vi "Pump Out Selection.vi"(6 "Module Type":enum16{"Feed Module", "Pump Module"}(ring), 7 "Calibration Y Intercept":dbl, 8 "error in (no error)":errorcluster, 9 "Calibration Slope":dbl, 10 "Speed":dbl, 11 "Pump Settings In":T1={"Output Device"=enum."Default", "Masterflex"={"VISA resource name"="", "Simulated?"=FALSE, "Pump Number"=0.0, "Reverse?"=FALSE}, "Ismatech"={"VISA resource name"="", "Simulated?"=FALSE, "Pump Number"=0.0, "Reverse?"=FALSE}, "Ismatech 3 Channel Settings"={"VISA resource name"="", "Pump Number"=1, "Channel Number"=0, "Simulated?"=TRUE, "Reverse?"=FALSE}, "VICI Settings"={"VISA resource name"="", "Pump ID"="", "Pump Head Vol"=0.0, "Reverse?"=FALSE, "Simulated?"=FALSE}, "Tacmina Settings"={"Analog DAQ Task"="", "Digital DAQ Task"=""}, "KNF SIMDOS Settings"={"VISA resource name"="", "Simulated?"=FALSE}, "ASIA Pump C"={"ASIA Pump #"=0, "channel"=0, "Simulated"=FALSE}, "FLOM Settings"={"VISA resource name"="", "Simulated?"=FALSE, "Pump Number"=0.0}, "SSI PR/LD Settings"={"VISA resource name"="", "Simulated?"=FALSE}, "SSI P40 Settings"={"VISA resource name"="", "Simulated?"=FALSE}, "Masterflex 75211 Settings"={"Analog DAQ Task"="", "Digital DAQ Task"=""}} {"Ismatech 3 Channel Settings"."Channel Number" min=0 max=3; "Ismatech 3 Channel Settings"."Pump Number" min=1; "Masterflex"."Pump Number" min=1.0 max=20.0 step=1.0; "Ismatech"."Pump Number" min=1.0 max=20.0 step=1.0; "ASIA Pump C"."channel" min=-1 max=1 step=1}) -> (0 "error out":errorcluster, 2 "Connection Error":bool, 3 "Pump Settings Out":T1={"Output Device"=enum."Default", "Masterflex"={"VISA resource name"="", "Simulated?"=FALSE, "Pump Number"=0.0, "Reverse?"=FALSE}, "Ismatech"={"VISA resource name"="", "Simulated?"=FALSE, "Pump Number"=0.0, "Reverse?"=FALSE}, "Ismatech 3 Channel Settings"={"VISA resource name"="", "Pump Number"=1, "Channel Number"=0, "Simulated?"=TRUE, "Reverse?"=FALSE}, "VICI Settings"={"VISA resource name"="", "Pump ID"="", "Pump Head Vol"=0.0, "Reverse?"=FALSE, "Simulated?"=FALSE}, "Tacmina Settings"={"Analog DAQ Task"="", "Digital DAQ Task"=""}, "KNF SIMDOS Settings"={"VISA resource name"="", "Simulated?"=FALSE}, "ASIA Pump C"={"ASIA Pump #"=0, "channel"=0, "Simulated"=FALSE}, "FLOM Settings"={"VISA resource name"="", "Simulated?"=FALSE, "Pump Number"=0.0}, "SSI PR/LD Settings"={"VISA resource name"="", "Simulated?"=FALSE}, "SSI P40 Settings"={"VISA resource name"="", "Simulated?"=FALSE}, "Masterflex 75211 Settings"={"Analog DAQ Task"="", "Digital DAQ Task"=""}} {"Ismatech 3 Channel Settings"."Channel Number" min=0 max=3; "Ismatech 3 Channel Settings"."Pump Number" min=1; "Masterflex"."Pump Number" min=1.0 max=20.0 step=1.0; "Ismatech"."Pump Number" min=1.0 max=20.0 step=1.0; "ASIA Pump C"."channel" min=-1 max=1 step=1})   [LabVIEW 2018, in "Pump Module.lvlib" / "Pump Module Engine.lvlib"]
uses:
  Pump Module Engine.lvlib
  Pump Settings Cluster.ctl
  Measure Instrument/PID 2 Output Enum.ctl
  Masterflex 7550-30/Controls/Settings Cluster.ctl
  Ismatec ISM 831C/Controls/Ismatech ISM831C Settings Cluster.ctl
  Ismatec 78001/Ismatec 4083.ctl
  VICI M50 Party Mode/Settings Cluster.ctl
  Tacmina QI/Tacmina QI DAQ Setting.ctl
  KNF Pump/Settings Cluster plus SIMDOS.ctl
  ASIA Pump/Pump Settings.ctl
  FLOM Pump/Settings Cluster.ctl
  SSI PR Class/SSI PR or LD Settings Cluster.ctl
  Masterflex 75211/Masterflex 75211 DAQ Setting.ctl
  Ismatec ISM 831C/Ismatec ISM 831C.lvlib
  Masterflex 7550-30/Masterflex 7550-30.lvlib
  VICI M50 Party Mode/VICI M6 M50 Party Mode.lvlib
  Tacmina QI/Tacmina QI.lvlib
  KNF Pump/KNF SIMDOS.lvlib
  ASIA Pump.lvlib
  FLOM Pump/FLOM Pump.lvlib
  SSI PR Class/SSI PR or LD Pump.lvlib
  Masterflex 75211/Masterflex 75211.lvlib
  SSI PR Class/SSI P40 Pump.lvlib
  Ismatec 78001/Ismatec 4308.lvlib
  Pump Module.lvlib
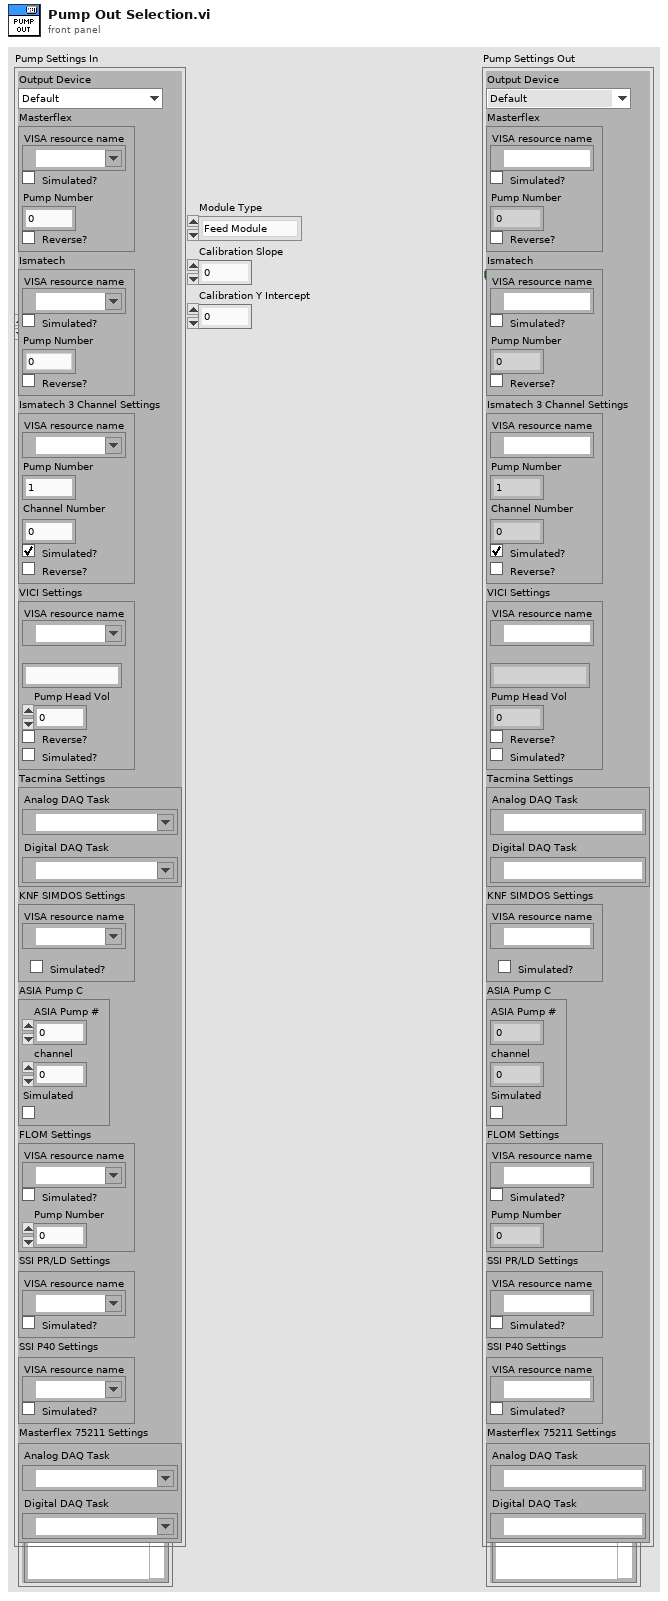
[diagram p1: front panel]
types:
  T1 = typedef "Pump Module.lvlib/Pump Settings Cluster.ctl" = cluster{"Output Device":T2, "Masterflex":T3, "Ismatech":T4, "Ismatech 3 Channel Settings":T5, "VICI Settings":T6, "Tacmina Settings":T7, "KNF SIMDOS Settings":T8, "ASIA Pump C":T9, "FLOM Settings":T10, "SSI PR/LD Settings":T11, "SSI P40 Settings":T11, "Masterflex 75211 Settings":T12}
  T2 = typedef "PID 2 Output Enum.ctl" = enum16{"Default", "Ismatec ISM 4308", "Ismatec ISM 831C", "Masterflex 7550-30", "VICI M6", "VICI M50", "Tacmina QI", "KNF SIMDOS", "ASIA Type C", "FLOM UI-22-11", "SSI PR/LD", "SSI P40", "Masterflex 75211-70"}
  T3 = typedef "Masterflex 7550-30.lvlib/Settings Cluster.ctl" = cluster{"VISA resource name":refnum<visa-resource-name>, "Simulated?":bool, "Pump Number":dbl, "Reverse?":bool}
  T4 = typedef "Ismatec ISM 831C.lvlib/Ismatech ISM831C Settings Cluster.ctl" = cluster{"VISA resource name":refnum<visa-resource-name>, "Simulated?":bool, "Pump Number":dbl, "Reverse?":bool}
  T5 = typedef "Ismatec 4308.lvlib/Ismatec 4083.ctl" = cluster{"VISA resource name":refnum<visa-resource-name>, "Pump Number":i16, "Channel Number":i16, "Simulated?":bool, "Reverse?":bool}
  T6 = typedef "VICI M6 M50 Party Mode.lvlib/Settings Cluster.ctl" = cluster{"VISA resource name":refnum<visa-resource-name>, "Pump ID":string, "Pump Head Vol":dbl, "Reverse?":bool, "Simulated?":bool}
  T7 = typedef "Tacmina QI.lvlib/Tacmina QI DAQ Setting.ctl" = cluster{"Analog DAQ Task":refnum<k21>, "Digital DAQ Task":refnum<k21>}
  T8 = typedef "KNF SIMDOS.lvlib/Settings Cluster plus SIMDOS.ctl" = cluster{"VISA resource name":refnum<visa-resource-name>, "Simulated?":bool}
  T9 = typedef "ASIA Pump.lvlib/Pump Settings.ctl" = cluster{"ASIA Pump #":i32, "channel":i32, "Simulated":bool}
  T10 = typedef "FLOM Pump.lvlib/Settings Cluster.ctl" = cluster{"VISA resource name":refnum<visa-resource-name>, "Simulated?":bool, "Pump Number":dbl}
  T11 = typedef "SSI PR or LD Pump.lvlib/SSI PR or LD Settings Cluster.ctl" = cluster{"VISA resource name":refnum<visa-resource-name>, "Simulated?":bool}
  T12 = typedef "Masterflex 75211.lvlib/Masterflex 75211 DAQ Setting.ctl" = cluster{"Analog DAQ Task":refnum<k21>, "Digital DAQ Task":refnum<k21>}
  T13 = typedef "SSI P40 Pump.lvlib/SSI P40 Settings Cluster.ctl" = cluster{"VISA resource name":refnum<visa-resource-name>, "Simulated?":bool}
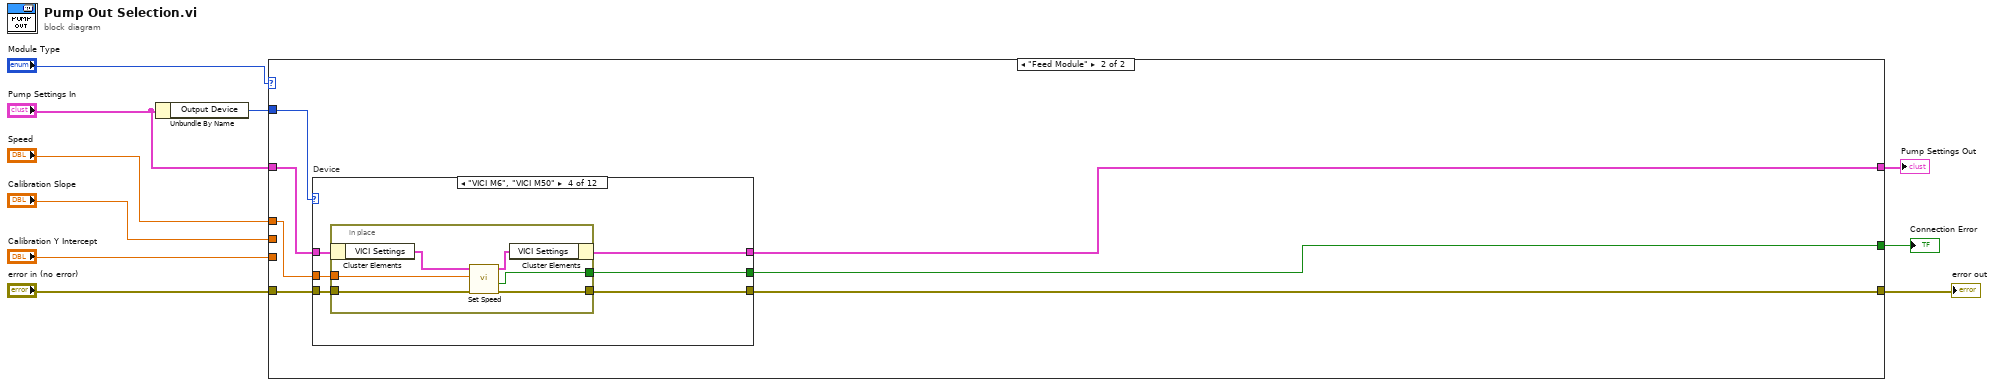
[diagram p0: block diagram]
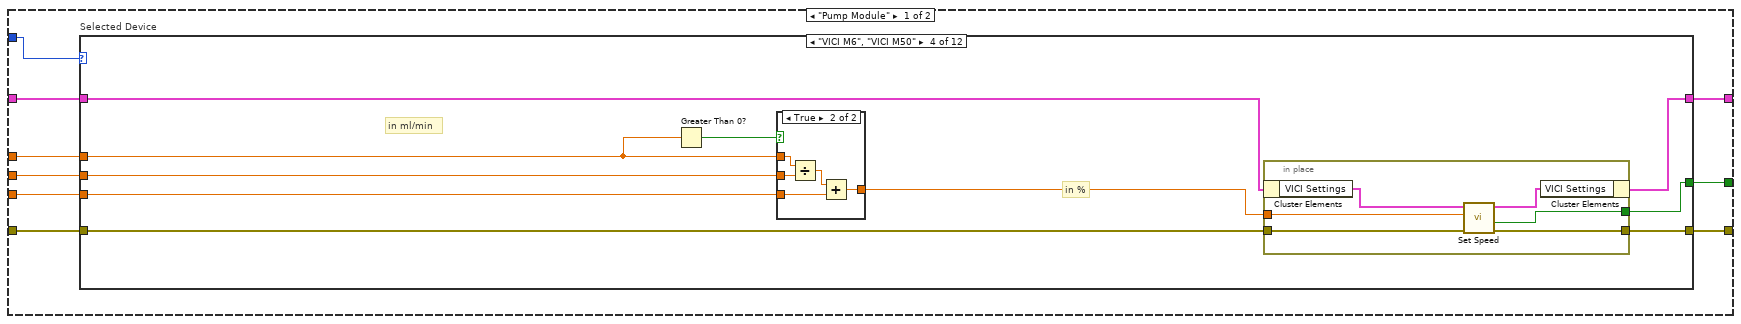
[diagram p2: hidden frame]
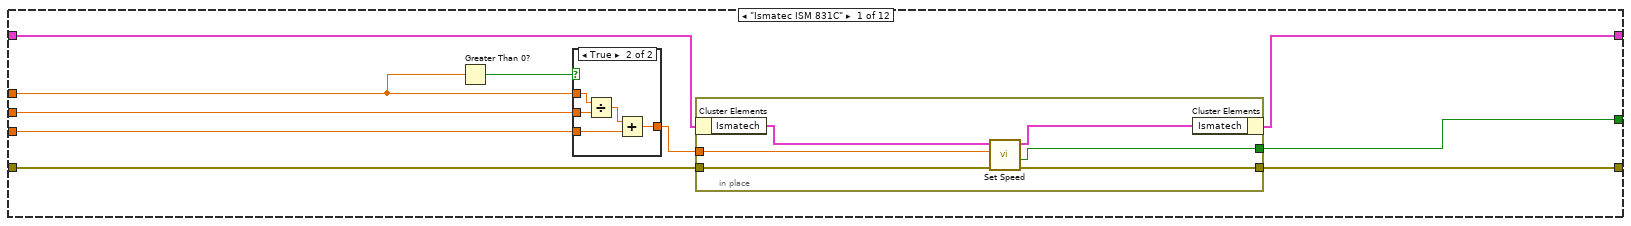
[diagram p3: hidden frame]
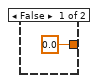
[diagram p4: hidden frame]
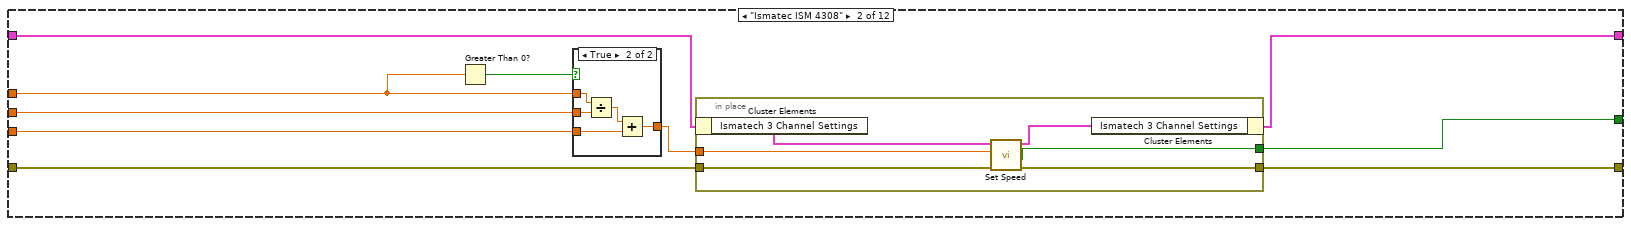
[diagram p5: hidden frame]
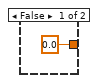
[diagram p6: hidden frame]
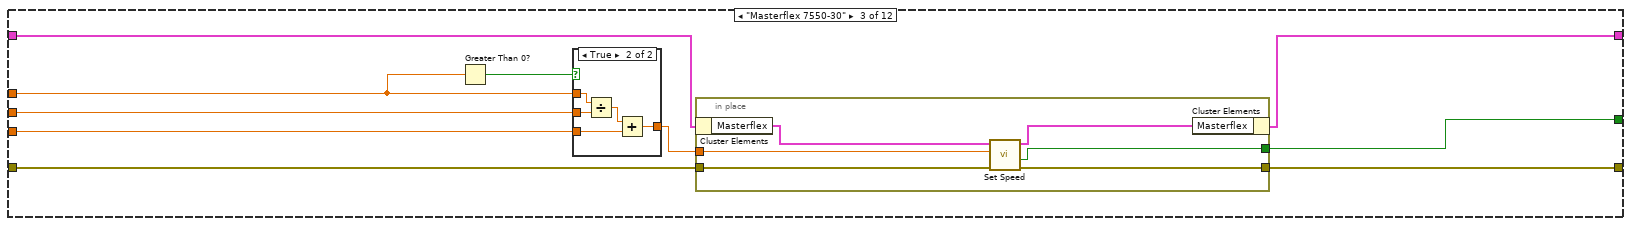
[diagram p7: hidden frame]
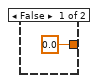
[diagram p8: hidden frame]
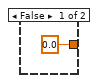
[diagram p9: hidden frame]
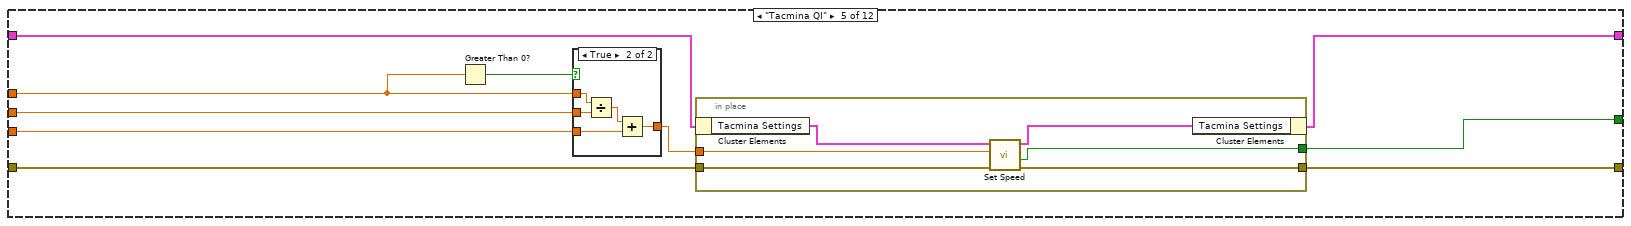
[diagram p10: hidden frame]
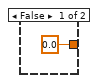
[diagram p11: hidden frame]
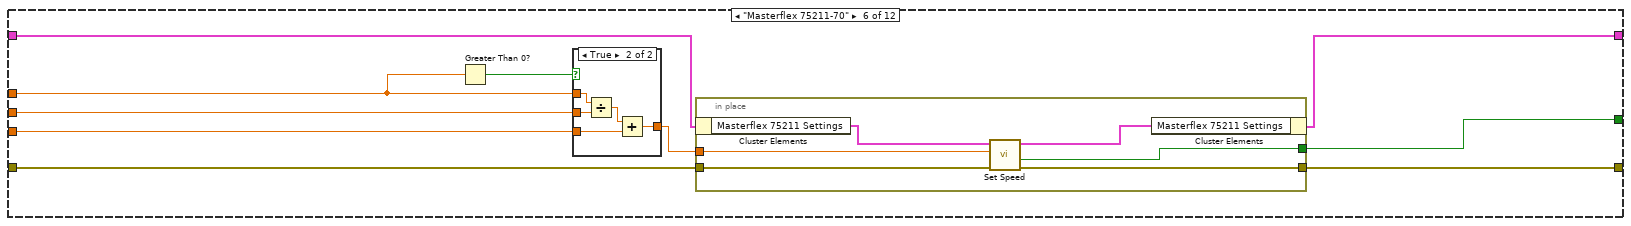
[diagram p12: hidden frame]
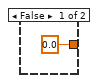
[diagram p13: hidden frame]
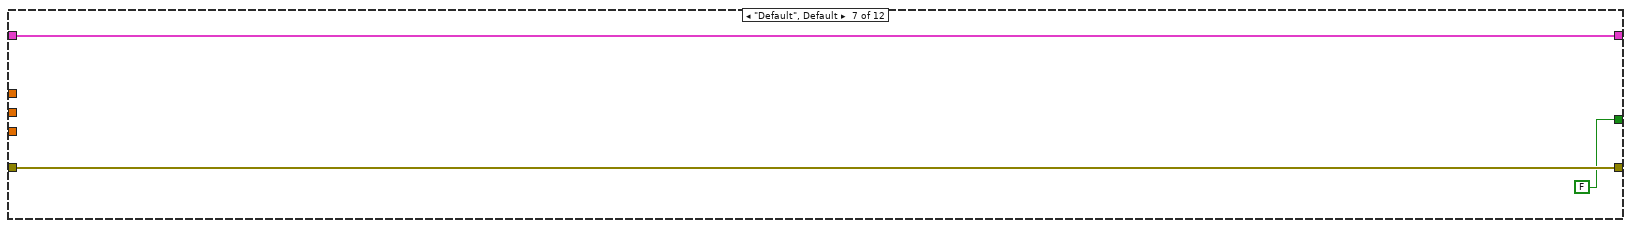
[diagram p14: hidden frame]
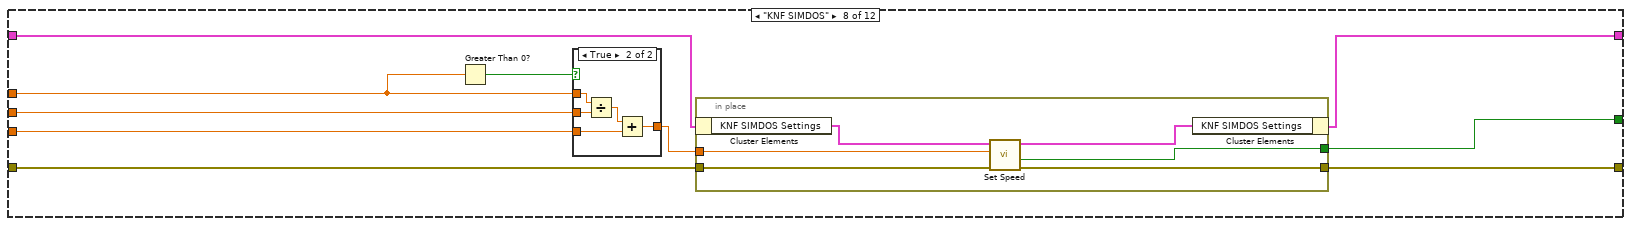
[diagram p15: hidden frame]
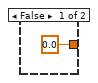
[diagram p16: hidden frame]
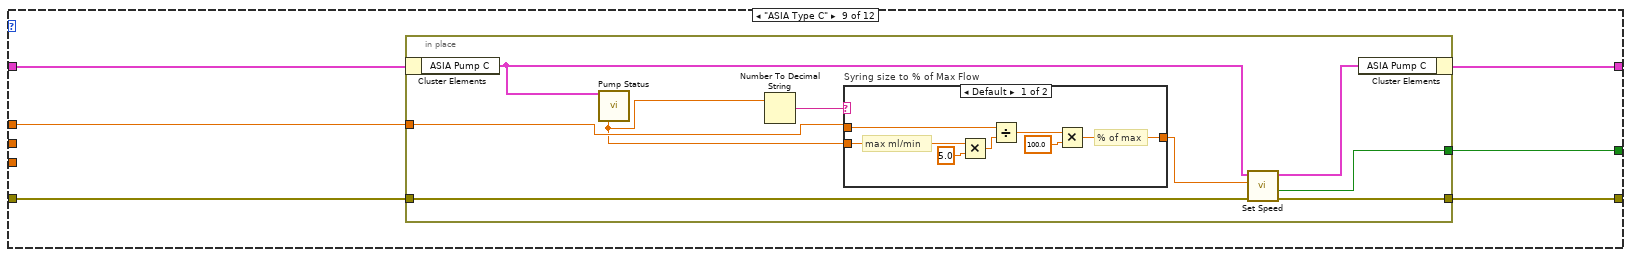
[diagram p17: hidden frame]
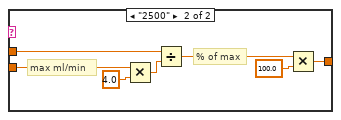
[diagram p18: hidden frame]
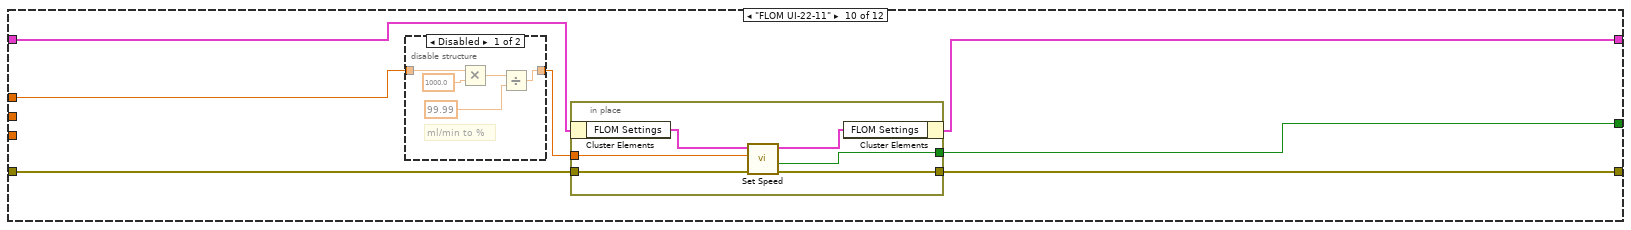
[diagram p19: hidden frame]
diagram:
  n1 = Unbundle By Name("Pump Settings In") -> ("Output Device"=w5:T2)
  n2 = case shown="\"Feed Module\"" "Module Type" {
    tunnel: [w19 w251] -> w10
    tunnel: [w18 w250] -> w9
    tunnel: "error in (no error)" -> [w17 w254]
    tunnel: "Speed" -> [w16 w253]
    tunnel: [w15 w252] -> w3
    tunnel: w5 -> [w14 w255]
    tunnel: "Calibration Slope" -> [w13 _]
    tunnel: "Calibration Y Intercept" -> [w12 _]
    tunnel: "Pump Settings In" -> [w11 w249]
    frame "Pump Module" {
      n3 = case "Selected Device" shown="\"VICI M6\", \"VICI M50\"" w14 {
        tunnel: w16 -> [w23 w45 w69 w91 w113 w135 _ w160 w179 w208 w230 w242]
        tunnel: w17 -> [w29 w51 w73 w95 w117 w139 w154 w164 w182 w212 w228 w240]
        tunnel: [w28 w50 w72 w94 w116 w138 w154 w163 w181 w210 w229 w241] -> w18
        tunnel: [w20 w42 w64 w86 w108 w130 w152 w155 w177 w206 w225 w237] -> w15
        tunnel: [w27 w49 w71 w93 w115 w137 FALSE ("Connection Error") w162 w180 w211 w227 w239] -> w19
        tunnel: w13 -> [w25 w47 w67 w90 w112 w134 _ w159 _ _ _ _]
        tunnel: w12 -> [w26 w48 w68 w88 w111 w133 _ w158 _ _ _ _]
        tunnel: w11 -> [w21 w43 w65 w87 w109 w131 w152 w156 w178 w207 w226 w238]
        frame "Ismatec ISM 831C" {
          n4 = Greater Than 0?(x=w23) -> (x > 0?=w22:bool)
          n5 = case shown="True" w22 {
            tunnel: w26 -> [_ w40]
            tunnel: w25 -> [_ w39]
            tunnel: w23 -> [_ w38]
            tunnel: [0.0 w37] -> w24
            frame False {
            }
            frame True {
              n6 = Divide(x=w38, y=w39) -> (x/y=w41:dbl)
              n7 = Add(x=w41, y=w40) -> (x+y=w37:dbl)
            }
          }
          n8 = in-place {
            in-place-border: w29 -> [w35]
            in-place-border: [w34] -> w28
            in-place-border: [w33] -> w27
            in-place-border: w24 -> [w32]
            n9 = in-place-cluster #1(w21) -> ("Ismatech"=w31:T4)
            n10 = call "Set Speed.vi"("error in (no error)"=w35, "Speed (%)"=w32, "Ismatech Settings In"=w31) -> ("error out"=w34:errorcluster, "Connection Error"=w33:bool, "Ismatech Settings Out"=w30:T4)  [unwired: 6 in]
            n11 = in-place-cluster #1("Ismatech"=w30) -> (w20:T1)
          }
        }
        frame "Ismatec ISM 4308" {
          n12 = Greater Than 0?(x=w45) -> (x > 0?=w44:bool)
          n13 = case shown="True" w44 {
            tunnel: w48 -> [_ w62]
            tunnel: w47 -> [_ w61]
            tunnel: w45 -> [_ w60]
            tunnel: [0.0 w59] -> w46
            frame False {
            }
            frame True {
              n14 = Divide(x=w60, y=w61) -> (x/y=w63:dbl)
              n15 = Add(x=w63, y=w62) -> (x+y=w59:dbl)
            }
          }
          n16 = in-place {
            in-place-border: w51 -> [w55]
            in-place-border: [w54] -> w50
            in-place-border: [w53] -> w49
            in-place-border: w46 -> [w56]
            n17 = in-place-cluster #2(w43) -> ("Ismatech 3 Channel Settings"=w57:T5)
            n18 = call "Set Speed.vi"("error in (no error)"=w55, "Speed (%)"=w56, "Ismatech 3 Channel Settings In"=w57) -> ("error out"=w54:errorcluster, "Connection Error"=w53:bool, "Ismatech 3 Channel Settings Out"=w52:T5)  [unwired: 5 in, 1 out]
            n19 = in-place-cluster #2("Ismatech 3 Channel Settings"=w52) -> (w42:T1)
          }
        }
        frame "Masterflex 7550-30" {
          n20 = Greater Than 0?(x=w69) -> (x > 0?=w70:bool)
          n21 = case shown="True" w70 {
            tunnel: w68 -> [_ w84]
            tunnel: w67 -> [_ w83]
            tunnel: w69 -> [_ w82]
            tunnel: [0.0 w81] -> w66
            frame False {
            }
            frame True {
              n22 = Divide(x=w82, y=w83) -> (x/y=w85:dbl)
              n23 = Add(x=w85, y=w84) -> (x+y=w81:dbl)
            }
          }
          n24 = in-place {
            in-place-border: w73 -> [w79]
            in-place-border: [w78] -> w72
            in-place-border: [w77] -> w71
            in-place-border: w66 -> [w76]
            n25 = in-place-cluster #3(w65) -> ("Masterflex"=w75:T3)
            n26 = call "Set Speed.vi"("error in (no error)"=w79, "speed"=w76, "Masterflex Settings in"=w75) -> ("error out"=w78:errorcluster, "Connection Error"=w77:bool, "Masterflex Settings out"=w74:T3)  [unwired: 6 in]
            n27 = in-place-cluster #3("Masterflex"=w74) -> (w64:T1)
          }
        }
        frame "VICI M6", "VICI M50" {
          # "in ml/min"
          # "in %"
          n28 = Greater Than 0?(x=w91) -> (x > 0?=w92:bool)
          n29 = case shown="True" w92 {
            tunnel: w88 -> [_ w106]
            tunnel: w90 -> [_ w105]
            tunnel: w91 -> [_ w104]
            tunnel: [0.0 w103] -> w89
            frame False {
            }
            frame True {
              n30 = Divide(x=w104, y=w105) -> (x/y=w107:dbl)
              n31 = Add(x=w107, y=w106) -> (x+y=w103:dbl)
            }
          }
          n32 = in-place {
            in-place-border: w95 -> [w101]
            in-place-border: [w100] -> w94
            in-place-border: [w99] -> w93
            in-place-border: w89 -> [w98]
            n33 = in-place-cluster #4(w87) -> ("VICI Settings"=w96:T6)
            n34 = call "Set Speed.vi"("error in (no error)"=w101, "Flow Rate (mL/min)"=w98, "VICI Settings In"=w96) -> ("error out"=w100:errorcluster, "Connection Error"=w99:bool, "VICI Settings Out"=w97:T6)  [unwired: 6 in]
            n35 = in-place-cluster #4("VICI Settings"=w97) -> (w86:T1)
          }
        }
        frame "Tacmina QI" {
          n36 = Greater Than 0?(x=w113) -> (x > 0?=w114:bool)
          n37 = case shown="True" w114 {
            tunnel: w111 -> [_ w128]
            tunnel: w112 -> [_ w127]
            tunnel: w113 -> [_ w126]
            tunnel: [0.0 w125] -> w110
            frame False {
            }
            frame True {
              n38 = Divide(x=w126, y=w127) -> (x/y=w129:dbl)
              n39 = Add(x=w129, y=w128) -> (x+y=w125:dbl)
            }
          }
          n40 = in-place {
            in-place-border: w117 -> [w123]
            in-place-border: [w122] -> w116
            in-place-border: [w121] -> w115
            in-place-border: w110 -> [w120]
            n41 = in-place-cluster #5(w109) -> ("Tacmina Settings"=w119:T7)
            n42 = call "Set Speed.vi"("error in"=w123, "Pump %"=w120, "Tacmina Settings in"=w119) -> ("error out"=w122:errorcluster, "Connection Error"=w121:bool, "Tacmina Settings out"=w118:T7)  [unwired: 6 in]
            n43 = in-place-cluster #5("Tacmina Settings"=w118) -> (w108:T1)
          }
        }
        frame "Masterflex 75211-70" {
          n44 = Greater Than 0?(x=w135) -> (x > 0?=w136:bool)
          n45 = case shown="True" w136 {
            tunnel: w133 -> [_ w150]
            tunnel: w134 -> [_ w149]
            tunnel: w135 -> [_ w148]
            tunnel: [0.0 w147] -> w132
            frame False {
            }
            frame True {
              n46 = Divide(x=w148, y=w149) -> (x/y=w151:dbl)
              n47 = Add(x=w151, y=w150) -> (x+y=w147:dbl)
            }
          }
          n48 = in-place {
            in-place-border: w139 -> [w140]
            in-place-border: [w142] -> w138
            in-place-border: [w143] -> w137
            in-place-border: w132 -> [w141]
            n49 = in-place-cluster #6(w131) -> ("Masterflex 75211 Settings"=w145:T12)
            n50 = call "Set Speed.vi"("error in"=w140, "Pump %"=w141, "Masterflex 75211 Settings"=w145) -> ("error out"=w142:errorcluster, "Connection Error"=w143:bool, "Masterflex 75211 Settings 2"=w144:T12)  [unwired: 6 in]
            n51 = in-place-cluster #6("Masterflex 75211 Settings"=w144) -> (w130:T1)
          }
        }
        frame "Default", Default {
        }
        frame "KNF SIMDOS" {
          n52 = Greater Than 0?(x=w160) -> (x > 0?=w161:bool)
          n53 = case shown="True" w161 {
            tunnel: w158 -> [_ w175]
            tunnel: w159 -> [_ w174]
            tunnel: w160 -> [_ w173]
            tunnel: [0.0 w172] -> w157
            frame False {
            }
            frame True {
              n54 = Divide(x=w173, y=w174) -> (x/y=w176:dbl)
              n55 = Add(x=w176, y=w175) -> (x+y=w172:dbl)
            }
          }
          n56 = in-place {
            in-place-border: w164 -> [w170]
            in-place-border: [w169] -> w163
            in-place-border: [w168] -> w162
            in-place-border: w157 -> [w167]
            n57 = in-place-cluster #7(w156) -> ("KNF SIMDOS Settings"=w166:T8)
            n58 = call "Set Speed.vi"("error in (no error)"=w170, "FlowRate"=w167, "KNF Settings In"=w166) -> ("error out"=w169:errorcluster, "Connection Error"=w168:bool, "KNF Settings Out"=w165:T8)  [unwired: 6 in]
            n59 = in-place-cluster #7("KNF SIMDOS Settings"=w165) -> (w155:T1)
          }
        }
        frame "ASIA Type C" {
          n60 = in-place {
            in-place-border: w182 -> [w191]
            in-place-border: [w190] -> w181
            in-place-border: [w189] -> w180
            in-place-border: w179 -> [w188]
            n61 = in-place-cluster #8(w178) -> ("ASIA Pump C"=w183:T9)
            n62 = call "Pump Status.vi"("ASIA Pump C Settings in"=w183) -> ("syringeSize (ml)"=w185:sgl)  [unwired: 6 in, 8 out]
            n63 = Number To Decimal String(number=w185) -> (decimal integer string=w187:string)  [unwired: 1 in]
            n64 = case "Syring size to % of Max Flow" shown="Default" w187 {
              tunnel: w185 -> [w197 w201]
              tunnel: w188 -> [w196 w200]
              tunnel: [w192 w199] -> w186
              frame Default {
                # "% of max"
                # "max ml/min"
                n65 = Multiply(x=w197, y=5.0) -> (x*y=w195:dbl)
                n66 = Divide(x=w196, y=w195) -> (x/y=w194:dbl)
                n67 = Multiply(x=w194, y=100.0) -> (x*y=w192:dbl)
              }
              frame "2500" {
                # "% of max"
                # "max ml/min"
                n68 = Multiply(x=w201, y=4.0) -> (x*y=w204:dbl)
                n69 = Divide(x=w200, y=w204) -> (x/y=w203:dbl)
                n70 = Multiply(x=w203, y=100.0) -> (x*y=w199:dbl)
              }
            }
            n71 = call "Set Speed.vi"("error in (no error)"=w191, "Pump %"=w186, "ASIA Pump C Settings in"=w183) -> ("error out"=w190:errorcluster, "Connection Error"=w189:bool, "ASIA Pump C Settings out"=w184:T9)  [unwired: 6 in]
            n72 = in-place-cluster #8("ASIA Pump C"=w184) -> (w177:T1)
          }
        }
        frame "FLOM UI-22-11" {
          n73 = disable-structure shown="Disabled" {
            disable-tunnel: [w222 w224] -> w209
            disable-tunnel: w208 -> [w220 w224]
            frame Disabled {
              # "ml/min to %"
              n74 = Multiply(x=w220, y=1000.0) -> (x*y=w219:dbl)
              n75 = Divide(x=w219, y=99.99) -> (x/y=w222:dbl)
            }
            frame Enabled {
            }
          }
          n76 = in-place {
            in-place-border: w212 -> [w218]
            in-place-border: [w217] -> w211
            in-place-border: [w216] -> w210
            in-place-border: w209 -> [w215]
            n77 = in-place-cluster #9(w207) -> ("FLOM Settings"=w213:T10)
            n78 = call "Set Speed.vi"("error in (no error)"=w218, "speed"=w215, "FLOM Settings in"=w213) -> ("error out"=w216:errorcluster, "Connection Error"=w217:bool, "FLOM Settings out"=w214:T10)  [unwired: 6 in]
            n79 = in-place-cluster #9("FLOM Settings"=w214) -> (w206:T1)
          }
        }
        frame "SSI PR/LD" {
          n80 = in-place {
            in-place-border: w230 -> [w236]
            in-place-border: [w235] -> w229
            in-place-border: w228 -> [w234]
            in-place-border: [w233] -> w227
            n81 = in-place-cluster #10(w226) -> ("SSI PR/LD Settings"=w231:T11)
            n82 = call "Set Speed.vi"("error in (no error)"=w234, "speed (ml/min)"=w236, "SSI PR Settings In"=w231) -> ("error out"=w235:errorcluster, "Connection Error"=w233:bool, "SSI PR Settings Out"=w232:T11)  [unwired: 6 in]
            n83 = in-place-cluster #10("SSI PR/LD Settings"=w232) -> (w225:T1)
          }
        }
        frame "SSI P40" {
          n84 = in-place {
            in-place-border: w242 -> [w247]
            in-place-border: [w245] -> w241
            in-place-border: w240 -> [w246]
            in-place-border: [w244] -> w239
            n85 = in-place-cluster #11(w238) -> ("SSI P40 Settings"=w248:T11)
            n86 = call "Set Speed P40.vi"("error in (no error)"=w246, "speed (ml/min)"=w247, "SSI P40 Settings In"=w248) -> ("error out"=w245:errorcluster, "Connection Error"=w244:bool, "SSI P40 Settings Out"=w243:T13)  [unwired: 6 in]
            n87 = in-place-cluster #11("SSI P40 Settings"=w243) -> (w237:T1)
          }
        }
      }
    }
    frame "Feed Module" {
      n88 = case "Device" shown="\"VICI M6\", \"VICI M50\"" w255 {
        tunnel: w253 -> [w259 w271 w283 w297 w309 w321 _ w336 w348 w359 w370 w382]
        tunnel: w254 -> [w261 w273 w285 w296 w308 w320 w329 w335 w345 w360 w372 w384]
        tunnel: [w260 w272 w284 w295 w307 w319 w329 w334 w347 w357 w371 w383] -> w250
        tunnel: w249 -> [w257 w269 w281 w293 w305 w317 w330 w332 w344 w356 w368 w380]
        tunnel: [w256 w268 w280 w292 w304 w316 w330 w331 w343 w355 w367 w379] -> w252
        tunnel: [w258 w270 w282 w294 w306 w318 FALSE ("Connection Error") w333 w346 w358 w369 w381] -> w251
        frame "Ismatec ISM 831C" {
          n89 = in-place {
            in-place-border: w261 -> [w267]
            in-place-border: [w266] -> w260
            in-place-border: w257 -> [_]
            in-place-border: w259 -> [w265]
            in-place-border: [w264] -> w258
            n90 = in-place-cluster #12(w257) -> ("Ismatech"=w262:T4)
            n91 = call "Set Speed.vi"("error in (no error)"=w267, "Speed (%)"=w265, "Ismatech Settings In"=w262) -> ("error out"=w266:errorcluster, "Connection Error"=w264:bool, "Ismatech Settings Out"=w263:T4)  [unwired: 6 in]
            n92 = in-place-cluster #12("Ismatech"=w263) -> (w256:T1)
          }
        }
        frame "Ismatec ISM 4308" {
          n93 = in-place {
            in-place-border: w273 -> [w279]
            in-place-border: [w278] -> w272
            in-place-border: w271 -> [w275]
            in-place-border: [w274] -> w270
            n94 = in-place-cluster #13(w269) -> ("Ismatech 3 Channel Settings"=w276:T5)
            n95 = call "Set Speed.vi"("error in (no error)"=w279, "Speed (%)"=w275, "Ismatech 3 Channel Settings In"=w276) -> ("error out"=w278:errorcluster, "Connection Error"=w274:bool, "Ismatech 3 Channel Settings Out"=w277:T5)  [unwired: 5 in, 1 out]
            n96 = in-place-cluster #13("Ismatech 3 Channel Settings"=w277) -> (w268:T1)
          }
        }
        frame "Masterflex 7550-30" {
          n97 = in-place {
            in-place-border: w285 -> [w291]
            in-place-border: [w290] -> w284
            in-place-border: w283 -> [w289]
            in-place-border: [w288] -> w282
            n98 = in-place-cluster #14(w281) -> ("Masterflex"=w287:T3)
            n99 = call "Set Speed.vi"("error in (no error)"=w291, "speed"=w289, "Masterflex Settings in"=w287) -> ("error out"=w290:errorcluster, "Connection Error"=w288:bool, "Masterflex Settings out"=w286:T3)  [unwired: 6 in]
            n100 = in-place-cluster #14("Masterflex"=w286) -> (w280:T1)
          }
        }
        frame "VICI M6", "VICI M50" {
          n101 = in-place {
            in-place-border: w297 -> [w303]
            in-place-border: w296 -> [w302]
            in-place-border: [w301] -> w295
            in-place-border: [w300] -> w294
            n102 = in-place-cluster #15(w293) -> ("VICI Settings"=w298:T6)
            n103 = call "Set Speed.vi"("error in (no error)"=w302, "Flow Rate (mL/min)"=w303, "VICI Settings In"=w298) -> ("error out"=w301:errorcluster, "Connection Error"=w300:bool, "VICI Settings Out"=w299:T6)  [unwired: 6 in]
            n104 = in-place-cluster #15("VICI Settings"=w299) -> (w292:T1)
          }
        }
        frame "Tacmina QI" {
          n105 = in-place {
            in-place-border: w309 -> [w315]
            in-place-border: w308 -> [w314]
            in-place-border: [w313] -> w307
            in-place-border: [w312] -> w306
            n106 = in-place-cluster #16(w305) -> ("Tacmina Settings"=w310:T7)
            n107 = call "Set Speed.vi"("error in"=w314, "Pump %"=w315, "Tacmina Settings in"=w310) -> ("error out"=w313:errorcluster, "Connection Error"=w312:bool, "Tacmina Settings out"=w311:T7)  [unwired: 6 in]
            n108 = in-place-cluster #16("Tacmina Settings"=w311) -> (w304:T1)
          }
        }
        frame "Masterflex 75211-70" {
          n109 = in-place {
            in-place-border: w321 -> [w325]
            in-place-border: w320 -> [w326]
            in-place-border: [w322] -> w319
            in-place-border: [w323] -> w318
            n110 = in-place-cluster #17(w317) -> ("Masterflex 75211 Settings"=w327:T12)
            n111 = call "Set Speed.vi"("error in"=w326, "Pump %"=w325, "Masterflex 75211 Settings"=w327) -> ("error out"=w322:errorcluster, "Connection Error"=w323:bool, "Masterflex 75211 Settings 2"=w324:T12)  [unwired: 6 in]
            n112 = in-place-cluster #17("Masterflex 75211 Settings"=w324) -> (w316:T1)
          }
        }
        frame "Default", Default {
        }
        frame "KNF SIMDOS" {
          n113 = in-place {
            in-place-border: w336 -> [w342]
            in-place-border: w335 -> [w341]
            in-place-border: [w340] -> w334
            in-place-border: [w339] -> w333
            n114 = in-place-cluster #18(w332) -> ("KNF SIMDOS Settings"=w338:T8)
            n115 = call "Set Speed.vi"("error in (no error)"=w341, "FlowRate"=w342, "KNF Settings In"=w338) -> ("error out"=w340:errorcluster, "Connection Error"=w339:bool, "KNF Settings Out"=w337:T8)  [unwired: 6 in]
            n116 = in-place-cluster #18("KNF SIMDOS Settings"=w337) -> (w331:T1)
          }
        }
        frame "ASIA Type C" {
          n117 = in-place {
            in-place-border: w348 -> [w354]
            in-place-border: [w353] -> w347
            in-place-border: [w352] -> w346
            in-place-border: w345 -> [w351]
            n118 = in-place-cluster #19(w344) -> ("ASIA Pump C"=w350:T9)
            n119 = call "Set Speed.vi"("error in (no error)"=w351, "Pump %"=w354, "ASIA Pump C Settings in"=w350) -> ("error out"=w353:errorcluster, "Connection Error"=w352:bool, "ASIA Pump C Settings out"=w349:T9)  [unwired: 6 in]
            n120 = in-place-cluster #19("ASIA Pump C"=w349) -> (w343:T1)
          }
        }
        frame "FLOM UI-22-11" {
          n121 = in-place {
            in-place-border: w360 -> [w366]
            in-place-border: w359 -> [w365]
            in-place-border: [w364] -> w358
            in-place-border: [w363] -> w357
            n122 = in-place-cluster #20(w356) -> ("FLOM Settings"=w361:T10)
            n123 = call "Set Speed.vi"("error in (no error)"=w366, "speed"=w365, "FLOM Settings in"=w361) -> ("error out"=w363:errorcluster, "Connection Error"=w364:bool, "FLOM Settings out"=w362:T10)  [unwired: 6 in]
            n124 = in-place-cluster #20("FLOM Settings"=w362) -> (w355:T1)
          }
        }
        frame "SSI PR/LD" {
          n125 = in-place {
            in-place-border: w372 -> [w378]
            in-place-border: [w377] -> w371
            in-place-border: w370 -> [w376]
            in-place-border: [w375] -> w369
            n126 = in-place-cluster #21(w368) -> ("SSI PR/LD Settings"=w374:T11)
            n127 = call "Set Speed.vi"("error in (no error)"=w378, "speed (ml/min)"=w376, "SSI PR Settings In"=w374) -> ("error out"=w377:errorcluster, "Connection Error"=w375:bool, "SSI PR Settings Out"=w373:T11)  [unwired: 6 in]
            n128 = in-place-cluster #21("SSI PR/LD Settings"=w373) -> (w367:T1)
          }
        }
        frame "SSI P40" {
          n129 = in-place {
            in-place-border: w384 -> [w388]
            in-place-border: [w385] -> w383
            in-place-border: w382 -> [w389]
            in-place-border: [w386] -> w381
            n130 = in-place-cluster #22(w380) -> ("SSI P40 Settings"=w390:T11)
            n131 = call "Set Speed P40.vi"("error in (no error)"=w388, "speed (ml/min)"=w389, "SSI P40 Settings In"=w390) -> ("error out"=w385:errorcluster, "Connection Error"=w386:bool, "SSI P40 Settings Out"=w387:T13)  [unwired: 6 in]
            n132 = in-place-cluster #22("SSI P40 Settings"=w387) -> (w379:T1)
          }
        }
      }
    }
  }
  "Connection Error" <- w10
  "error out" <- w9
  "Pump Settings Out" <- w3
